vi "SL TAGS Read Server Batch Tags.vi"(8 "error in (no error)":errorcluster, 11 "Tags In":T1[](array[typedef])) -> (0 "error out":errorcluster, 3 "Tags Out":T1[](array[typedef]))   [LabVIEW 2017, in "EEISysLink.lvclass"]
doc: "Will input an array of class tags and read thier values from the SystemLink server using Read Multiple for an efficient exchange. \n\nJames Tillett P.E.\nEndeavor Engineering Inc.\nwww.endeavoreng.com"
uses:
  EEISysLink.lvclass
  Controls/SL Tag.ctl
  <vilib>/Skyline/Tag/Wrapper/Wrapper_class/NI Skyline Tag.lvclass
  Controls/SL Tag Properties.ctl
  Controls/SL Tag Data Type.ctl
  Controls/SL Tag Interpolation Method.ctl
  Controls/SL Tag Unit of Measure.ctl
  Controls/SL Tag Type.ctl
  <vilib>/Skyline/Tag/Shared/typedefs/Tag Cluster.ctl
  <vilib>/Skyline/Tag/Shared/typedefs/DataType.ctl
  <vilib>/Skyline/Tag/Shared/NI Skyline Tag.lvlib
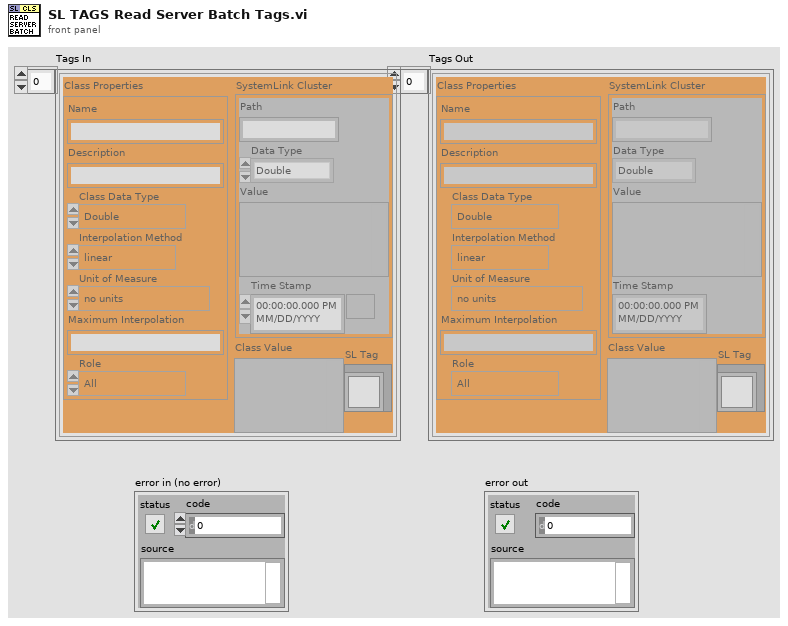
[diagram p1: front panel]
types:
  T1 = typedef "EEISysLink.lvclass/SL Tag.ctl" = cluster{"Class Properties":T2, "SL Tag":refnum<class "NI Skyline Tag.lvclass">, "SystemLink Cluster":T7, "Class Value":variant}
  T2 = typedef "EEISysLink.lvclass/SL Tag Properties.ctl" = cluster{"Class Data Type":T3, "Name":string, "Description":string, "Interpolation Method":T4, "Unit of Measure":T5, "Maximum Interpolation":string, "Role":T6}
  T3 = typedef "EEISysLink.lvclass/SL Tag Data Type.ctl" = enum16{"Double", "Integer", "String", "Boolean", "Waveform"}
  T4 = typedef "EEISysLink.lvclass/SL Tag Interpolation Method.ctl" = enum16{"linear", "pilinear", "step"}
  T5 = typedef "EEISysLink.lvclass/SL Tag Unit of Measure.ctl" = enum16{"no units", "Second", "Hour", "Minute", "Day", "Year", "Month", "Week", "Foot", "Yard", "Meter", "Centimeter", "Inch", "Mile", "Nautical Mile", "Miles per Hour", "Meters per second", "Square meter", "Cubic meter", "Cubic centimeter", "Cubic inch", "Liter", "Gallon", "Gallons dry US", "Gallon UK", "Percent", "Revolutions per minute", "Revolution", "Degree angle", "Astronomical Unit", "Atom", "Atomic mass", "Bar", "Byte", "C (speed of light)", "Curie", "Decibel", "Electron Volt", "Ounce", "Knot", "G", "Grade", "Are", "Hectare", "Faraday", "Franklin", "Gilbert", "Erg", "Lambert", "Maxwell", "Gauss", "Electron mass", "Kilogram force", "Pound force", "Rad", "Centiradian", "Sphere", "Mach", "Fluid Ounces", "Fluid Ounces UK", "Fahrenheit", "Celsius", "Kelvin", "Rankine", "Gram", "Kilogram", "Pound", "Short/US Ton", "Long/UK ton", "Metric ton", "Mole", "Pounds per square inch", "Inches water column", "Torr", "Millitorr", "Millimeter mercury", "Inches mercury", "Bar (2)", "Atmosphere", "Pascal", "Watt", "kiloWatt", "Horsepower", "Kilowatt Hour", "British thermal units", "Millions of BTU", "Ampere", "Candela", "Radian", "Steradian", "Bit", "Hertz", "Newton", "Joule", "Coulomb", "Volt", "Farad", "Ohm", "Siemens", "Weber", "Tesla", "Henry", "Lumen", "Lux", "Becqueral", "Gray", "Sievert", "Katal", "Angstrom", "Light Year", "Parsec", "Point", "Pixel", "Dyne", "Kilogram force (2)", "Pound force (2)", "Rem", "Rutherford", "Roentgen"}
  T6 = typedef "EEISysLink.lvclass/SL Tag Type.ctl" = enum16{"All", "Supervisor", "Worker"}
  T7 = typedef "NI Skyline Tag.lvlib/Tag Cluster.ctl" = cluster{"Path":string, "Data Type":T8, "Value":variant, "Time Stamp":timestamp}
  T8 = typedef "NI Skyline Tag.lvlib/DataType.ctl" = enum32{"Double", "Integer", "String"}
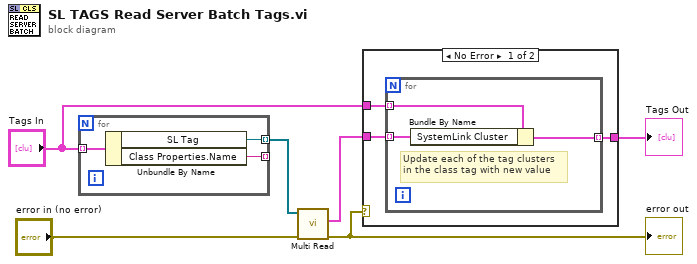
[diagram p0: block diagram]
diagram:
  n1 = for {
    tunnel: "Tags In" -> [w9] mode=indexing
    tunnel: [w8] -> w6 mode=indexing
    tunnel: [w7] -> _ mode=indexing
    n2 = Unbundle By Name(w9) -> ("SL Tag"=w8:refnum<class "NI Skyline Tag.lvclass">, "Class Properties.Name"=w7:string)
  }
  n3 = call <vilib>:"Multi Read.vi"("error in (no error)"="error in (no error)", "tags in"=w6) -> ("error out"=w1:errorcluster, "tag clusters"=w3:T7[])  [unwired: 7 in, 1 out]
  "error out" <- w1
  n4 = case shown="No Error" w1 {
    tunnel: "Tags In" -> [w12 w16]
    tunnel: w3 -> [w11 _]
    tunnel: [w10 w16] -> w2
    frame No Error {
      n5 = for {
        tunnel: w12 -> [w15] mode=indexing
        tunnel: w11 -> [w14] mode=indexing
        tunnel: [w13] -> w10 mode=indexing
        # "Update each of the tag clusters\nin the class tag with new value"
        n6 = Bundle By Name(cluster=w15, "SystemLink Cluster"=w14) -> (w13:T1)
      }
    }
    frame Error {
      # "If error then return unchanged"
    }
  }
  "Tags Out" <- w2
